vi "getForceStop.vi"(8 "error in (no error)":errorcluster, 11 "TaskMock in":refnum<class "TaskMock.lvclass">) -> (0 "error out":errorcluster, 2 "forceStop":refnum<notifier>, 3 "TaskMock out":refnum<class "TaskMock.lvclass">)   [LabVIEW 2023, in "TaskMock.lvclass"]
uses:
  TaskMock.lvclass
  TaskMock.lvclass/TaskMock.ctl
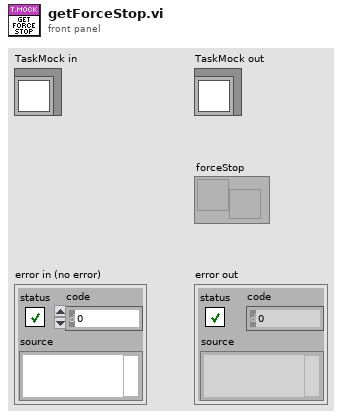
[diagram p1: front panel]
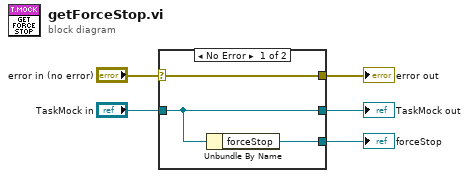
[diagram p0: block diagram]
diagram:
  n1 = case shown="No Error" "error in (no error)" {
    selector: "error in (no error)" -> [w8 w10]
    tunnel: [w8 w10] -> w4
    tunnel: [w7 w9] -> w2
    tunnel: "TaskMock in" -> [w7 w9]
    tunnel: [w6 _] -> w1
    frame No Error {
      n2 = Unbundle By Name(w7) -> ("forceStop"=w6:refnum<notifier>)
    }
    frame Error {
    }
  }
  "error out" <- w4
  "TaskMock out" <- w2
  "forceStop" <- w1
